vi "getTitleImage.vi"(3 "error in (no error)":errorcluster caption="错误输入（无错误）", 4 "story":T1) -> (0 "title":string, 1 "error out":errorcluster caption="错误输出", 2 "图片":picture)   [LabVIEW 2012]
panel:
  out "响应体":string
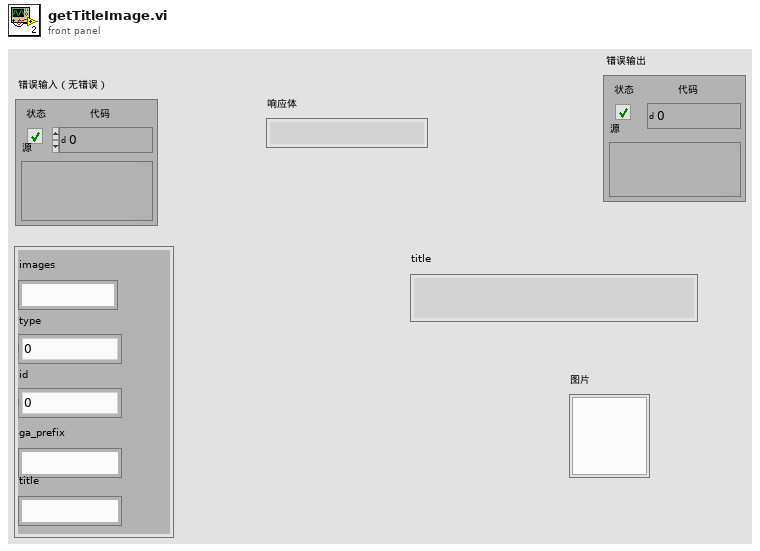
[diagram p1: front panel]
types:
  T1 = cluster{"images":string, "type":i32, "id":i64, "ga_prefix":string, "title":string}
  T2 = typedef "imagedata.ctl" = cluster{"image type":i32, "image depth":i32, "image":u8[], "mask":u8[], "colors":u32[], "Rectangle":cluster{"left":i16, "top":i16, "right":i16, "bottom":i16}}
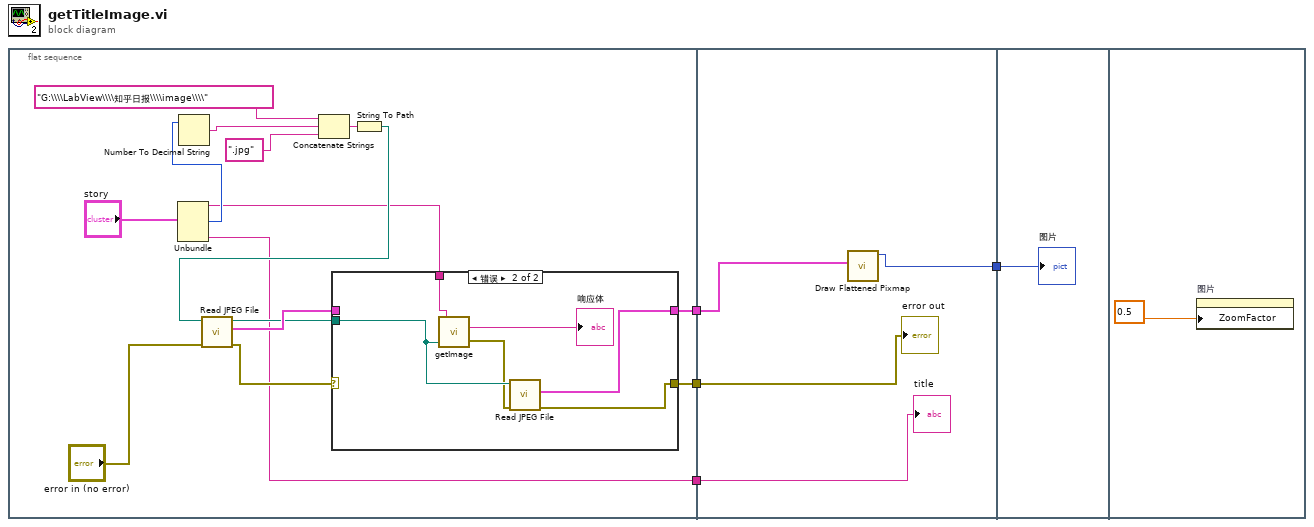
[diagram p0: block diagram]
diagram:
  n1 = flat-sequence {
    tunnel: [w10] -> w3
    tunnel: [w9] -> w2
    tunnel: [w5] -> w1
    tunnel: [w31] -> w4
    tunnel: w3 -> [w30]
    tunnel: w2 -> [w29]
    tunnel: w1 -> [w28]
    tunnel: w4 -> [w32]
    frame #0 {
      n2 = Unbundle("story") -> ("images"=w6:string, "id"=w18:i64, "title"=w5:string)  [unwired: 2 out]
      n3 = Number To Decimal String(number=w18) -> (decimal integer string=w14:string)  [unwired: 1 in]
      n4 = Concatenate Strings("G:\\\\LabView\\\\知乎日报\\\\image\\\\", w14, ".jpg") -> (w16:string)
      n5 = String To Path(string=w16) -> (path=w8:path)
      n6 = call <vilib>:"Read JPEG File.vi"("error in (no error)"="error in (no error)", "path to JPEG file"=w8) -> ("error out"=w12:errorcluster, "image data"=w11:T2, "path"=w7:path)  [unwired: 7 in]
      n7 = case shown="错误" w12 {
        selector: w12 -> [w20 _]
        tunnel: w11 -> [w21 _]
        tunnel: [w21 w23] -> w10
        tunnel: [w20 w22] -> w9
        tunnel: w7 -> [_ w25]
        tunnel: w6 -> [_ w27]
        frame No Error {
        }
        frame Error {
          n8 = call "getImage.vi"("路径"=w25, "URL"=w27) -> ("error out"=w24:errorcluster, "响应体"=→"响应体":string)  [unwired: 1 in]
          n9 = call <vilib>:"Read JPEG File.vi"("error in (no error)"=w24, "path to JPEG file"=w25) -> ("error out"=w22:errorcluster, "image data"=w23:T2)  [unwired: 7 in, 1 out]
        }
      }
    }
    frame #1 {
      n10 = call <vilib>:"Draw Flattened Pixmap.vi"("image data"=w30) -> ("new picture"=w31:picture)  [unwired: 8 in]
      "title" <- w28
      "error out" <- w29
    }
    frame #2 {
      "图片" <- w32
    }
    frame #3 {
      n11 = property on="图片" class="Pict"("ZoomFactor"=0.5) -> ()  [unwired: 2 in, 2 out]
    }
  }
